vi "Wellington2.vi"() -> ()   [LabVIEW 2009]
uses:
  <vilib>/NXT/Block Support/NXT_InputPort.ctl
  <vilib>/NXT/Block Support/NXT_ButtonSelector.ctl
  <vilib>/NXT/Subs/MotorOutput.ctl
  <vilib>/NXT/Dual Mode Library/Waits/Wait_Num.vi
  <vilib>/NXT/Dual Mode Library/Display/drawText.vi
  <vilib>/NXT/Dual Mode Library/Sensors/Light_On.vi
  <vilib>/NXT/Dual Mode Library/Sensors/readNXTButton.vi
  <vilib>/NXT/Dual Mode Library/Sensors/Touch_Pressed.vi
  <vilib>/NXT/Dual Mode Library/Sensors/Sound_dB.vi
  <vilib>/NXT/Dual Mode Library/Sensors/Sonar_cm.vi
  <vilib>/NXT/Subs/NXT_SteeringOutputPort.ctl
panel:
  out "Cor inicial":i16
  out "Verificacao":bool[](array[boolean])
  out "Toque":bool
  out "Visor":string
  out "Ruído":i16(slide) scale=0.0..100.0
  out "Luminosidade":i16
  out "Distância":i16
  out "Botao":bool
  # "O Mindstorms irá ficar no seguinte loop até que o botão central seja precionado:\nAciona os motores B e C para frente.\nMostrará os valores dos sensores na tela.\nCaso seja detectado: uma distância menor que 50cm, ou um ruído maior que 70dB, ou o sensor de toque seja precionado ou haja uma mudança de cor. O Mindstorms irá executar a seguinte rotina:\nIrá desligar os motores B e C.\nIrá ligar os motores B e C para trás e dará cinco voltas.\nSelecionará aleatoriamente um lado (direita/esquerda).\nEmitirá um som \"äleatório\".\nVirará 180 graus para o lado escolhido.\nE voltará ao loop."
  # "Configuração:\nOUT_A: GARRA\nOUT_B: RODA DA ESQUERDA\nOUT_C: RODA DA DIREITA\nIN_1: SENSOR DE TOQUE\nIN_2: SENSOR SONORO\nIN_3: SENSOR LUMINOSO\nIN_4: SENSOR ULTRA-SOM"
  # "1 - Distância menor que 50cm\n2 - Mudança de cor detectada\n3 - Ruído maior que 70dB\n4 - Toque precionado"
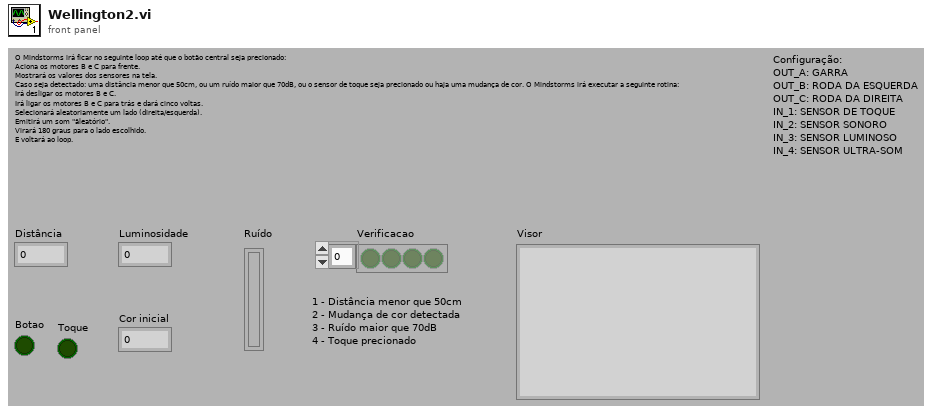
[diagram p1: front panel]
types:
  T1 = typedef "MotorOutput.ctl" = u8
  T2 = typedef "NXT_InputPort.ctl" = u8
  T3 = typedef "LVHSConnector.ctl" = cluster{"error":errorcluster, "address":string, "NXT #":i32, "Show Error":bool, "Connection":u16}
  T4 = typedef "NXT_ButtonSelector.ctl" = u16
  T5 = typedef "NXT_SteeringOutputPort.ctl" = u16
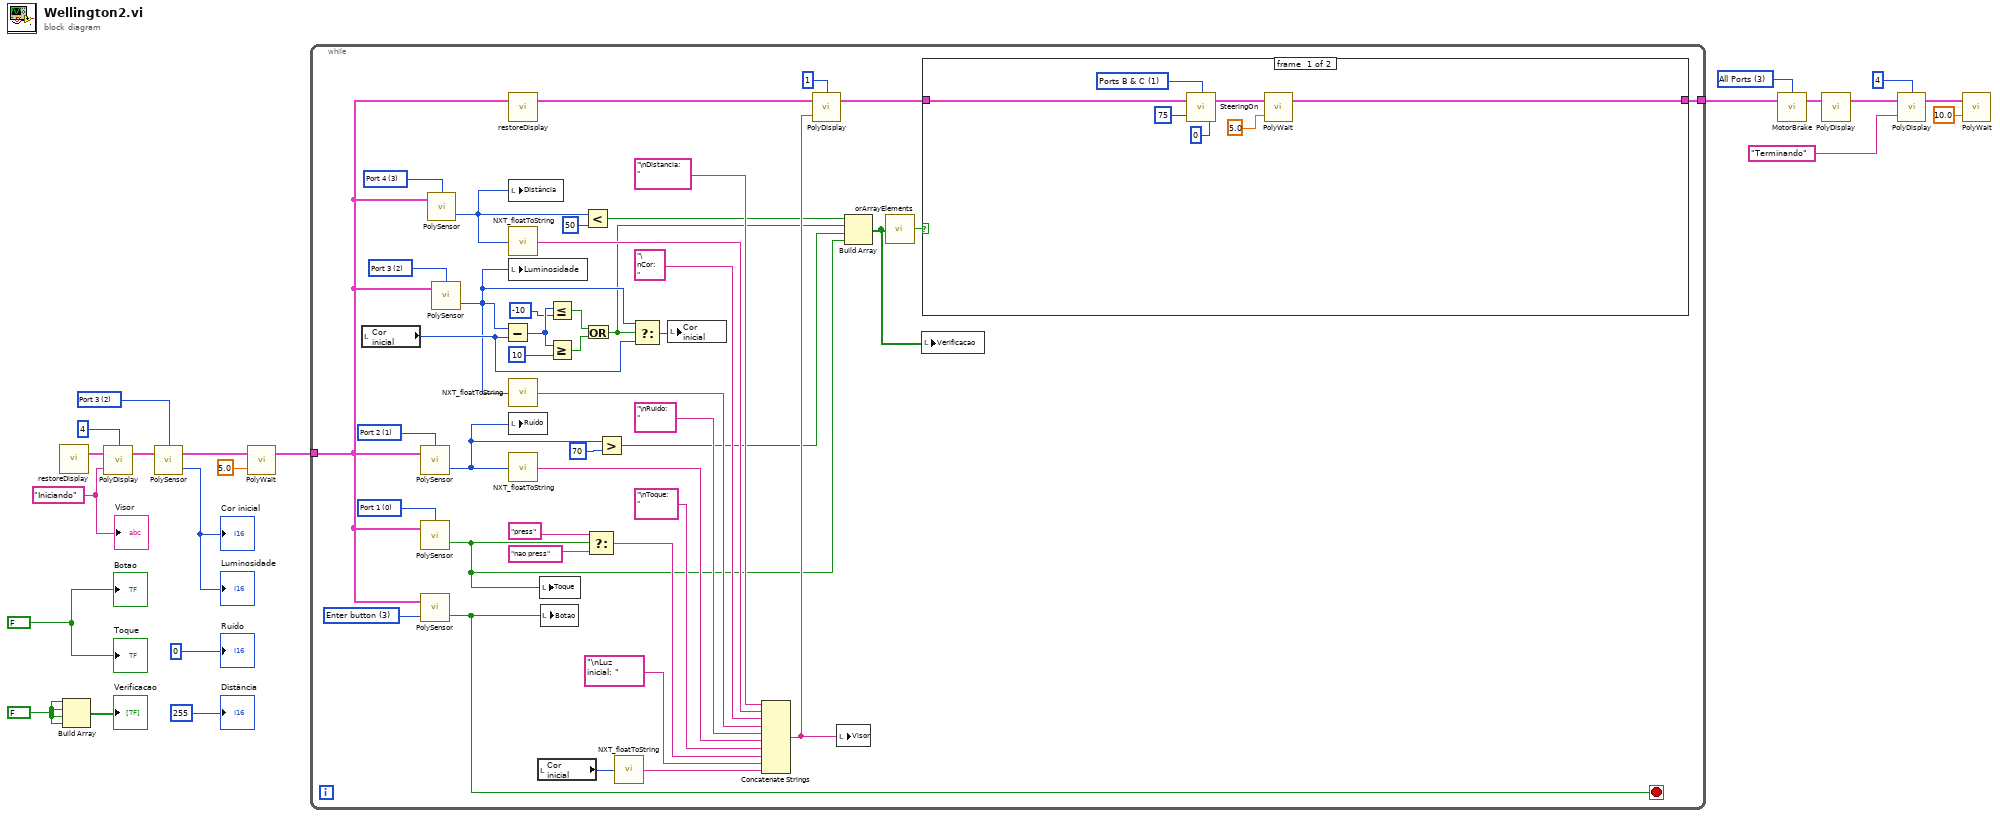
[diagram p0: block diagram]
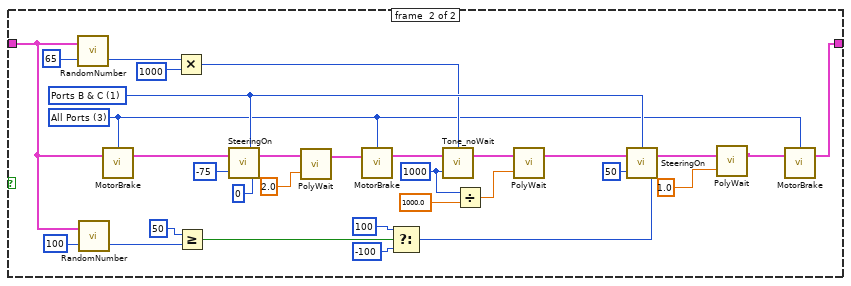
[diagram p2: hidden frame]
diagram:
  w2 = FALSE
  w14 = T1 3 items=["Port A", "Port B", "Port C", "All Ports"] ("Output Port (All Ports)")
  w10 = T2 2 items=["Port 1", "Port 2", "Port 3", "Port 4"] ("Input Port")
  w21 = "Iniciando"
  w20 = FALSE
  n1 = call <vilib>:"restoreDisplay.vi"() -> ("NXT"=w15:T3)  [unwired: 4 in]
  n2 = Build Array(w2, w2, w2, w2) -> (→"Verificacao":bool[])
  n3 = call-poly <vilib>:"PolyDisplay.vi"("Text"=w21, "NXT"=w15, "Line"=i16 4) -> ("NXT"=w7:T3)  [unwired: 1 in]
  n4 = call-poly <vilib>:"PolySensor.vi"("NXT"=w7, "Port (Port 3)"=w10) -> ("Scaled Value"=→"Luminosidade" →"Cor inicial":i16, "NXT"=w8:T3)  [unwired: 1 in]
  n5 = call-poly <vilib>:"PolyWait.vi"("Time (1 sec)"=sgl 5.0, "NXT"=w8) -> ("NXT"=w6:T3)  [unwired: 2 in]
  n6 = while {
    tunnel: w6 -> [w43]
    tunnel: [w42] -> w4
    stop <- w65 stop-if-true
    w48 = T4 3 items=["Enter button"=3, "Left button"=2, "Right button"=1] ("Button (Enter button)")
    w61 = T2 3 items=["Port 1", "Port 2", "Port 3", "Port 4"] ("Input Port")
    w62 = T2 2 items=["Port 1", "Port 2", "Port 3", "Port 4"] ("Input Port")
    w63 = T2 1 items=["Port 1", "Port 2", "Port 3", "Port 4"] ("Input Port")
    w64 = T2 0 items=["Port 1", "Port 2", "Port 3", "Port 4"] ("Input Port")
    n7 = local read "Cor inicial"() -> (w33:i16)
    n8 = call-poly <vilib>:"PolySensor.vi"("NXT"=w43, "Port (Port 2)"=w63) -> ("Sound (dB)"=w29:i16)  [unwired: 1 in, 1 out]
    n9 = call-poly <vilib>:"PolySensor.vi"("NXT"=w43, "Port (Port 1)"=w64) -> ("Yes / No"=w27:bool)  [unwired: 1 in, 1 out]
    n10 = call-poly <vilib>:"PolySensor.vi"("Button (Enter button)"=w48, "NXT"=w43) -> ("Yes/No"=w65:bool)  [unwired: 1 in, 1 out]
    n11 = call-poly <vilib>:"PolySensor.vi"("NXT"=w43, "Port (Port 4)"=w61) -> ("Distance (cm)"=w40:i16)  [unwired: 1 in, 1 out]
    n12 = call-poly <vilib>:"PolySensor.vi"("NXT"=w43, "Port (Port 3)"=w62) -> ("Scaled Value"=w32:i16)  [unwired: 1 in, 1 out]
    n13 = Subtract(x=w32, y=w33) -> (x-y=w24:i16)
    n14 = call <vilib>:"restoreDisplay.vi"("NXT"=w43) -> ("NXT"=w47:T3)  [unwired: 3 in]
    n15 = local write "Distância"(w40) -> ()
    n16 = call <vilib>:"NXT_floatToString.vi"("number"=w40) -> ("string"=w57:string)
    n17 = local write "Luminosidade"(w32) -> ()
    n18 = call <vilib>:"NXT_floatToString.vi"("number"=w32) -> ("string"=w55:string)
    n19 = local write "Ruído"(w29) -> ()
    n20 = call <vilib>:"NXT_floatToString.vi"("number"=w29) -> ("string"=w51:string)
    n21 = local read "Cor inicial"() -> (w46:i16)
    n22 = local write "Toque"(w27) -> ()
    n23 = local write "Botao"(w65) -> ()
    n24 = Less Or Equal?(x=w24, y=i16 -10) -> (x <= y?=w34:bool)
    n25 = Greater Or Equal?(x=w24, y=i16 10) -> (x >= y?=w35:bool)
    n26 = Less?(x=w40, y=i16 50) -> (x < y?=w38:bool)
    n27 = Or(x=w34, y=w35) -> (x .or. y?=w31:bool)
    n28 = Select(t="press", s=w27, f="nao press") -> (s? t:f=w53:string)
    n29 = Greater?(x=w29, y=i16 70) -> (0:w28:bool)
    n30 = call <vilib>:"NXT_floatToString.vi"("number"=w46) -> ("string"=w44:string)
    n31 = Select(t=w32, s=w31, f=w33) -> (s? t:f=w37:i16)
    n32 = local write "Cor inicial"(w37) -> ()
    n33 = Concatenate Strings("\nDistancia: ", w57, "\nCor: ", w55, "\nRuido: ", w51, "\nToque: ", w53, "\nLuz inicial: ", w44) -> (w49:string)
    n34 = call-poly <vilib>:"PolyDisplay.vi"("Text"=w49, "NXT"=w47, "Line"=i16 1) -> ("NXT"=w25:T3)  [unwired: 1 in]
    n35 = local write "Visor"(w49) -> ()
    n36 = Build Array(w38, w31, w28, w27) -> (w26:bool[])
    n37 = call <vilib>:"orArrayElements.vi"("Boolean Array"=w26) -> ("Logical OR"=w41:bool)
    n38 = local write "Verificacao"(w26) -> ()
    n39 = case shown="True" w41 {
      tunnel: w25 -> [w69 w100]
      tunnel: [w66 w75] -> w42
      frame #0 {
        w70 = T5 1 items=["Ports A & B", "Ports B & C", "Ports A & C"] ("Output Port")
        n40 = call <vilib>:"SteeringOn.vi"("Power (75)"=75, "Steering (100)"=0, "NXT"=w69, "Output Ports"=w70) -> ("NXT"=w67:T3)
        n41 = call-poly <vilib>:"PolyWait.vi"("Time (1 sec)"=sgl 5.0, "NXT"=w67) -> ("NXT"=w66:T3)  [unwired: 2 in]
      }
      frame #1 {
        w84 = u16 1000
        w82 = T1 3 items=["Port A", "Port B", "Port C", "All Ports"] ("Output Port (All Ports)")
        w99 = T5 1 items=["Ports A & B", "Ports B & C", "Ports A & C"] ("Output Port")
        n42 = call <vilib>:"RandomNumber.vi"("Max Value"=i16 65, "NXT"=w100) -> ("Random Number"=w95:u16)  [unwired: 1 in, 1 out]
        n43 = call <vilib>:"RandomNumber.vi"("Max Value"=i16 100, "NXT"=w100) -> ("Random Number"=w91:u16)  [unwired: 1 in, 1 out]
        n44 = call <vilib>:"MotorBrake.vi"("NXT"=w100, "Port (All Ports)"=w82) -> ("NXT"=w74:T3)  [unwired: 2 in]
        n45 = Multiply(x=w95, y=i16 1000) -> (x*y=w93:u16)
        n46 = Greater Or Equal?(x=i16 50, y=w91) -> (x >= y?=w90:bool)
        n47 = call <vilib>:"SteeringOn.vi"("Power (75)"=-75, "Steering (100)"=0, "NXT"=w74, "Output Ports"=w99) -> ("NXT"=w78:T3)
        n48 = call-poly <vilib>:"PolyWait.vi"("Time (1 sec)"=sgl 2.0, "NXT"=w78) -> ("NXT"=w79:T3)  [unwired: 2 in]
        n49 = call <vilib>:"MotorBrake.vi"("NXT"=w79, "Port (All Ports)"=w82) -> ("NXT"=w83:T3)  [unwired: 2 in]
        n50 = Select(t=100, s=w90, f=-100) -> (s? t:f=w92:i32)
        n51 = call <vilib>:"Tone_noWait.vi"("Duration (500 ms)"=w84, "NXT"=w83, "Tone (440 Hz)"=w93) -> ("NXT"=w97:T3)  [unwired: 1 in]
        n52 = Divide(x=w84, y=sgl 1000.0) -> (x/y=w86:sgl)
        n53 = call-poly <vilib>:"PolyWait.vi"("Time (1 sec)"=w86, "NXT"=w97) -> ("NXT"=w73:T3)  [unwired: 2 in]
        n54 = call <vilib>:"SteeringOn.vi"("Power (75)"=50, "Steering (100)"=w92, "NXT"=w73, "Output Ports"=w99) -> ("NXT"=w81:T3)
        n55 = call-poly <vilib>:"PolyWait.vi"("Time (1 sec)"=sgl 1.0, "NXT"=w81) -> ("NXT"=w80:T3)  [unwired: 2 in]
        n56 = call <vilib>:"MotorBrake.vi"("NXT"=w80, "Port (All Ports)"=w82) -> ("NXT"=w75:T3)  [unwired: 2 in]
      }
    }
  }
  n57 = call <vilib>:"MotorBrake.vi"("NXT"=w4, "Port (All Ports)"=w14) -> ("NXT"=w12:T3)  [unwired: 2 in]
  n58 = call-poly <vilib>:"PolyDisplay.vi"("NXT"=w12) -> ("NXT"=w18:T3)  [unwired: 3 in]
  n59 = call-poly <vilib>:"PolyDisplay.vi"("Text"="Terminando", "NXT"=w18, "Line"=i16 4) -> ("NXT"=w11:T3)  [unwired: 1 in]
  n60 = call-poly <vilib>:"PolyWait.vi"("Time (1 sec)"=sgl 10.0, "NXT"=w11) -> ()  [unwired: 2 in, 1 out]
  "Botao" <- w20
  "Distância" <- i16 255
  "Ruído" <- i16 0
  "Visor" <- w21
  "Toque" <- w20
